vi "read_y.vi"(8 "error in (no error)":errorcluster, 11 "GammaRegressor in":refnum<class "GammaRegressor.lvclass">) -> (0 "error out":errorcluster, 2 "y":dbl[](array[numeric]), 3 "GammaRegressor out":refnum<class "GammaRegressor.lvclass">)   [LabVIEW 2020, in "GammaRegressor.lvclass"]
uses:
  GammaRegressor.lvclass
  GammaRegressor.lvclass/GammaRegressor.ctl
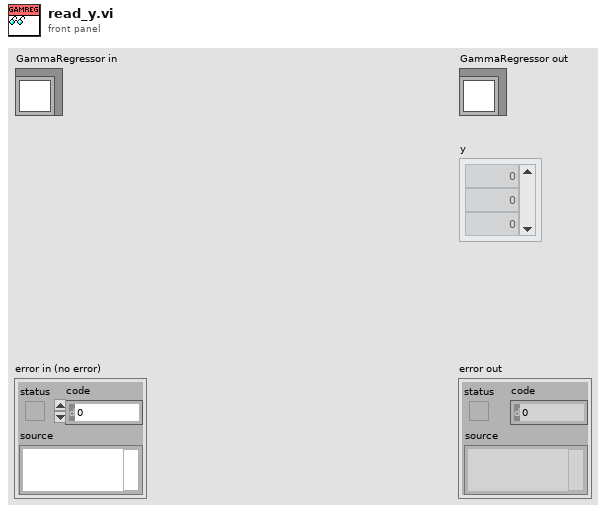
[diagram p1: front panel]
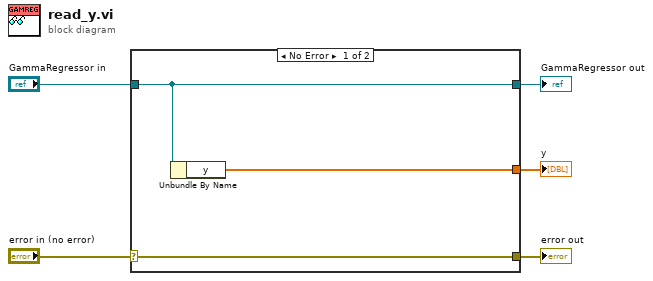
[diagram p0: block diagram]
diagram:
  n1 = case shown="No Error" "error in (no error)" {
    selector: "error in (no error)" -> [w8 w9]
    tunnel: [w8 w9] -> w4
    tunnel: [w7 w10] -> w2
    tunnel: "GammaRegressor in" -> [w7 w10]
    tunnel: [w6 _] -> w1
    frame No Error {
      n2 = Unbundle By Name(w7) -> ("y"=w6:dbl[])
    }
    frame Error {
    }
  }
  "error out" <- w4
  "GammaRegressor out" <- w2
  "y" <- w1
